vi "Computer Sequence Simulation Dialog.vi"(11 "Sequence Context":refnum<k7>) -> (0 "error out":errorcluster, 3 "Simulation Settings":T1)   [LabVIEW 2011]
doc: "Allows the user to specify which simulated motherboard components will fail."
panel:
  in  "Keyboard":bool
  in  "Video":bool
  in  "RAM":bool
  in  "CPU":bool
  in  "ROM":bool
  in  "Power":bool
  in  "OK":bool
  # "Select Simulated Components to Force Fail:"
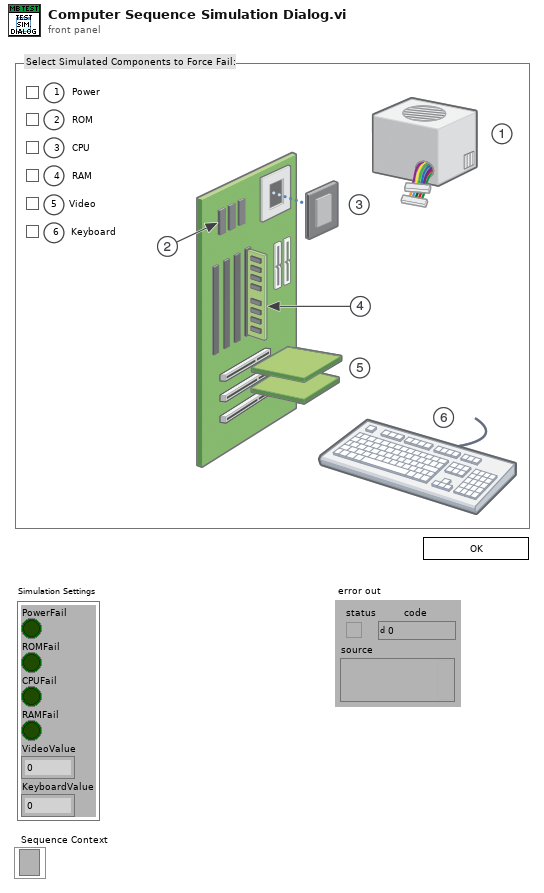
[diagram p1: front panel]
types:
  T1 = cluster{"PowerFail":bool, "ROMFail":bool, "CPUFail":bool, "RAMFail":bool, "VideoValue":dbl, "KeyboardValue":dbl}
  T2 = typedef "MotherboardTest - TestStand - Status Monitor.ctl" = cluster{"Sequence Context":refnum<k7>, "Execution":refnum<k7>, "Termination Monitor":refnum<k7>}
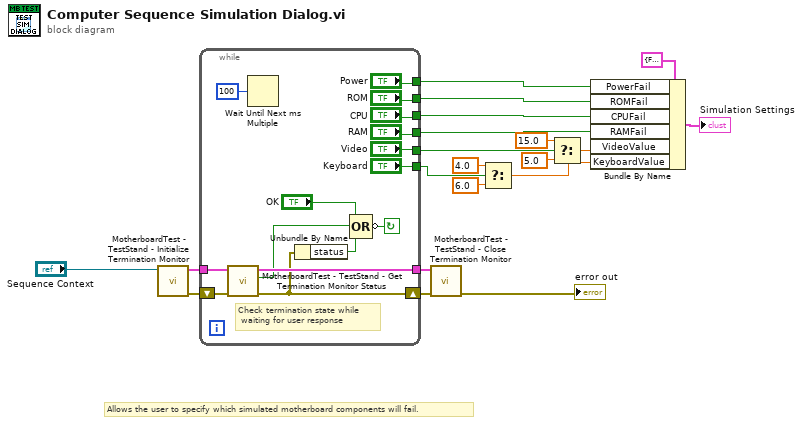
[diagram p0: block diagram]
diagram:
  # "Allows the user to specify which simulated motherboard components will fail."
  n1 = call "MotherboardTest - TestStand - Initialize Termination Monitor.vi"("Sequence Context In"="Sequence Context") -> ("error out"=w15:errorcluster, "Status Monitor Out"=w16:T2)  [unwired: 9 in]
  n2 = while {
    tunnel: w16 -> [w30]
    tunnel: [w29] -> w13
    shift-left: w15 -> [w31]
    shift-right: [w27] -> w14
    tunnel: ["Keyboard"] -> w9
    tunnel: ["Video"] -> w8
    tunnel: ["RAM"] -> w7
    tunnel: ["CPU"] -> w6
    tunnel: ["ROM"] -> w5
    tunnel: ["Power"] -> w4
    stop <- w34 continue-if-true
    # "Check termination state while\n waiting for user response"
    n3 = call "MotherboardTest - TestStand - Get Termination Monitor Status.vi"("error in (no error)"=w31, "Status Monitor In"=w30) -> ("error out"=w27:errorcluster, "Terminating or Aborting"=w28:bool, "Status Monitor Out"=w29:T2)  [unwired: 7 in]
    n4 = Wait Until Next ms Multiple(millisecond multiple=u32 100) -> ()  [unwired: 1 out]
    n5 = Unbundle By Name(w27) -> ("status"=w32:bool)
    n6 = Compound Arithmetic op=OR("OK", w28, w32) -> (invert w34:bool)
  }
  n7 = call "MotherboardTest - TestStand - Close Termination Monitor.vi"("error in (no error)"=w14, "Status Monitor In"=w13) -> ("error out"=→"error out":errorcluster)  [unwired: 9 in]
  n8 = Select(t=4.0, s=w9, f=6.0) -> (s? t:f=w10:dbl)
  n9 = Select(t=15.0, s=w8, f=5.0) -> (s? t:f=w11:dbl)
  n10 = Bundle By Name(cluster=T1 {"PowerFail"=FALSE, "ROMFail"=FALSE, "CPUFail"=FALSE, "RAMFail"=FALSE, "VideoValue"=5.0, "KeyboardValue"=6.0} ("Simulation Settings"), "PowerFail"=w4, "ROMFail"=w5, "CPUFail"=w6, "RAMFail"=w7, "VideoValue"=w11, "KeyboardValue"=w10) -> (→"Simulation Settings":T1)
